vi "constants.vi"() -> ()   [LabVIEW 2011, in "Diamond Universal Driver.lvlib"]
uses:
  Diamond Universal Driver.lvlib
panel:
  in  "version":string="0602"
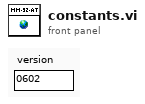
[diagram p1: front panel]
diagram:
